vi "PhRead.vi"(8 "error in":errorcluster, 10 "PhFilepath":path=path "\\\\lab14\\C/Users/bhuser/Documents/LabVIEW-BH/Jannis/Zeiss.ph") -> (0 "error out":errorcluster, 1 "MTclock[ns]":dbl, 2 "EventHeader":u32 format="%08x", 3 "PhotInfo64":T1[](array[typedef]) {"flags" max=3 format="%016b"; "rout_chan" step=1; "micro_time" step=1; "mtime" step=1})   [LabVIEW 2019]
doc: "This Vi demonstrates how a *.ph file in the Becker&Hickl propriety format can be read to a PhotInfo-cluster (structure).\n\ninfo@becker-hickl.com"
uses:
  SPC_Controls/SPC_PhotInfo64.ctl
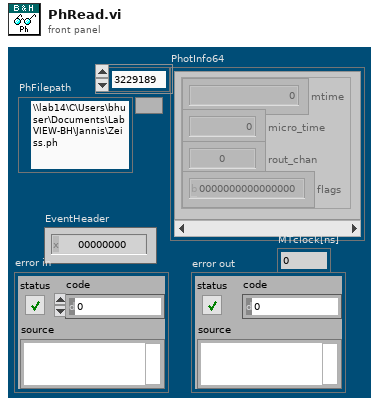
[diagram p1: front panel]
types:
  T1 = typedef "SPC_PhotInfo64.ctl" = cluster{"mtime":u64, "micro_time":u16, "rout_chan":u16, "flags":u16}
  T2 = enum16{"big-endian, network order", "native, host order", "little-endian"}
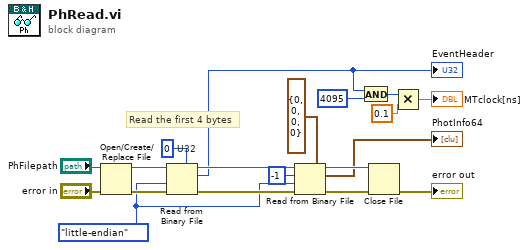
[diagram p0: block diagram]
diagram:
  w13 = T2."little-endian" ("byte order (0:big-endian, network order)")
  w18 = u32 0  # U32
  # "Read the first 4 bytes"
  n1 = Open/Create/Replace File(file path (use dialog)="PhFilepath", error in="error in") -> (refnum out=w16:refnum<file>, error out=w17:errorcluster)  [unwired: 4 in, 1 out]
  n2 = Read from Binary File(5:w18, 8:w17, 9:w13, 11:w16) -> (0:w14:errorcluster, 2:w5:u32, 3:w15:refnum<file>)  [unwired: 2 in, 1 out]
  "EventHeader" <- w5
  n3 = Read from Binary File(5:T1 {"mtime"=0, "micro_time"=0, "rout_chan"=0, "flags"=0} ("SPC_PhotInfo"), 8:w14, 9:w13, 10:-1 ("count (1)"), 11:w15) -> (0:w10:errorcluster, 2:→"PhotInfo64":T1[], 3:w11:refnum<file>)  [unwired: 1 in, 1 out]
  n4 = And(x=w5, y=u32 4095) -> (x .and. y?=w3:u32)
  n5 = Close File(refnum=w11, error in=w10) -> (error out=→"error out":errorcluster)  [unwired: 1 out]
  n6 = Multiply(x=w3, y=0.1 ("count (1)")) -> (x*y=→"MTclock[ns]":dbl)
